vi "Status Section.vi"(8 "error in (no error)":errorcluster, 11 "Node Ptr":T1 format="%.0x") -> (0 "error out":errorcluster)   [LabVIEW 2010, in "RefMem PtByPt Custom Device.lvlib"]
uses:
  RefMem PtByPt Custom Device.lvlib
  <vilib>/NI Veristand/Custom Device API/Custom Device Item Ref.ctl
  <vilib>/NI Veristand/Custom Device API/Custom Device API.lvlib
panel:
  in  "Header":cluster{"Section Name":string}={"Section Name"="Status Section"}
  in  "Description":string
  in  "Name":string
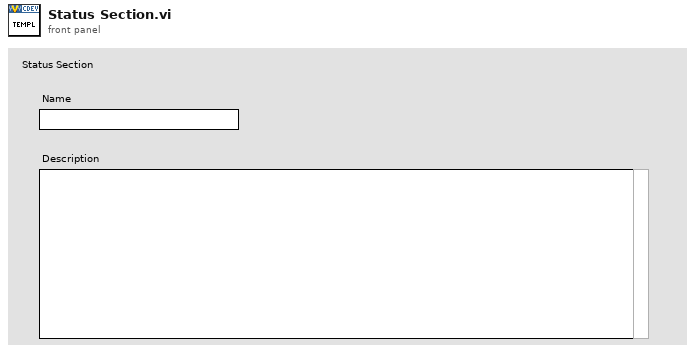
[diagram p1: front panel]
types:
  T1 = typedef "Custom Device API.lvlib/Custom Device Item Ref.ctl" = u64
  T2 = typedef "Custom Device API.lvlib/Custom Device Item Info.ctl" = cluster{"Name":string, "Is Channel":bool, "GUID":string}
  T3 = typedef "Custom Device API.lvlib/Custom Device Commands.ctl" = enum16{"Default", "Item renamed", "Shutdown", "Dynamic button pressed"}
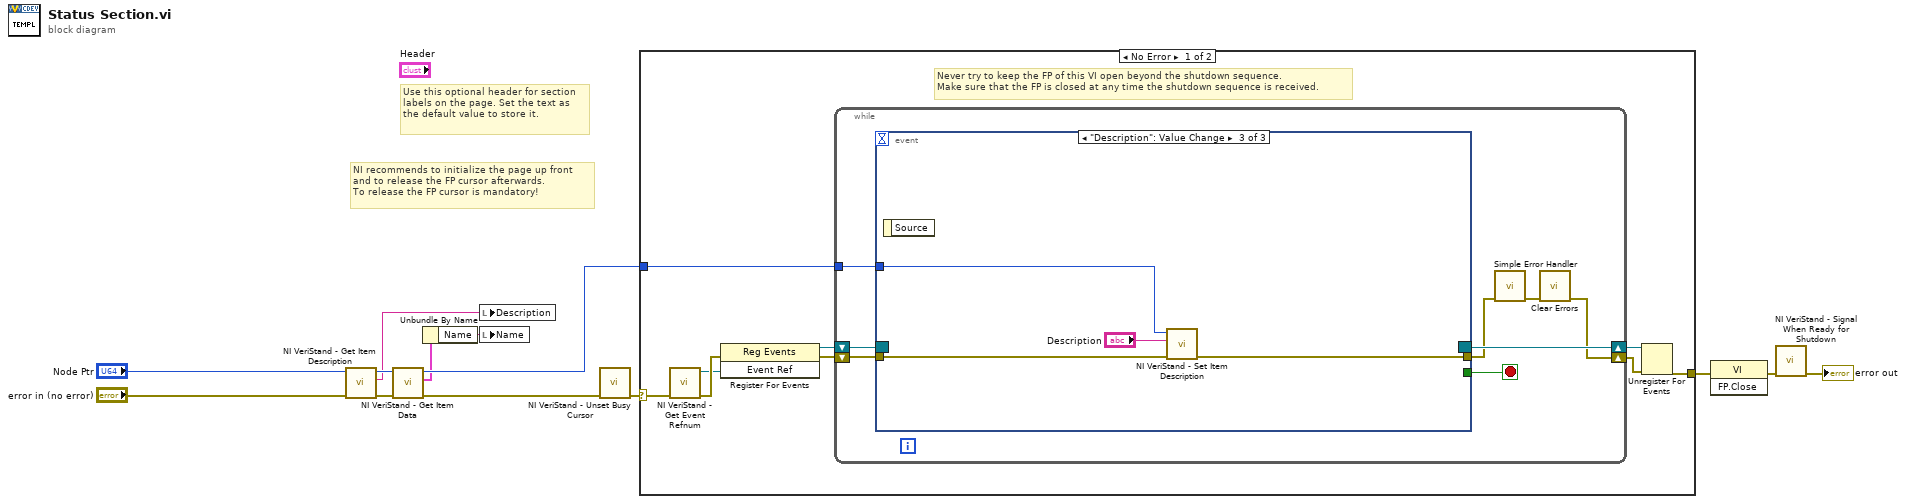
[diagram p0: block diagram]
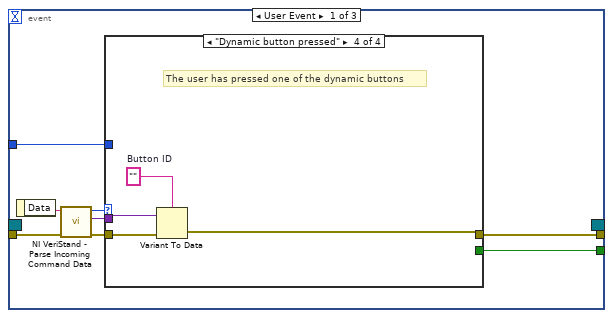
[diagram p2: hidden frame]
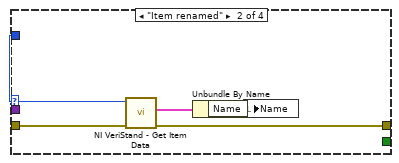
[diagram p4: hidden frame]
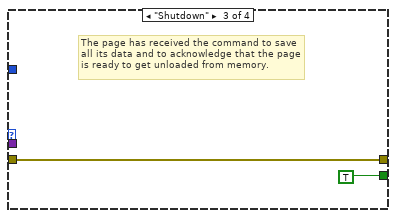
[diagram p5: hidden frame]
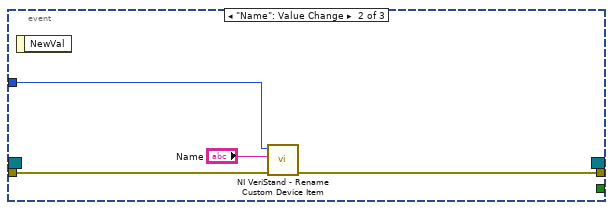
[diagram p6: hidden frame]
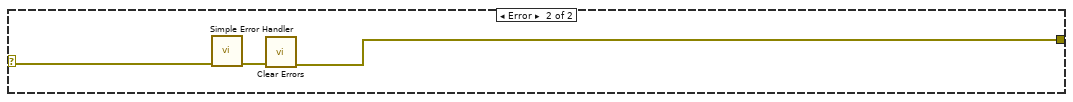
[diagram p7: hidden frame]
diagram:
  # "Use this optional header for section labels on the page. Set the text as the default value to store it."
  # "NI recommends to initialize the page up front\nand to release the FP cursor afterwards.\nTo release the FP cursor is mandatory!"
  n1 = call <vilib>:"NI VeriStand - Get Item Description.vi"("error in (no error)"="error in (no error)", "Item Ref in"="Node Ptr") -> ("error out"=w5:errorcluster, "Description"=w6:string, "Item Ref out"=w7:T1)  [unwired: 7 out]
  n2 = call <vilib>:"NI VeriStand - Get Item Data.vi"("error in (no error)"=w5, "Item Ref in"=w7) -> ("error out"=w10:errorcluster, "Item Info"=w4:T2, "Item Ref out"=w8:T1)  [unwired: 7 out]
  n3 = Unbundle By Name(w4) -> ("Name"=w3:string)
  n4 = local write "Description"(w6) -> ()
  n5 = local write "Name"(w3) -> ()
  n6 = call <vilib>:"NI VeriStand - Unset Busy Cursor.vi"("error in (no error)"=w10) -> ("error out"=w9:errorcluster)  [unwired: 10 out]
  n7 = case shown="No Error" w9 {
    selector: w9 -> [w14 w61]
    tunnel: [w19 w59] -> w13
    tunnel: w8 -> [w15 _]
    frame No Error {
      # "Never try to keep the FP of this VI open beyond the shutdown sequence.\nMake sure that the FP is closed at any time the shutdown sequence is received."
      n8 = call <vilib>:"NI VeriStand - Get Event Refnum.vi"("error in (no error)"=w14) -> ("error out"=w22:errorcluster, "Event Ref"=w18:refnum<user-event>)  [unwired: 9 out]
      n9 = register-events(error in=w22, w18) -> (reference out=w16:refnum<event-registration>, error out=w17:errorcluster)  [unwired: 1 in]
      n10 = while {
        tunnel: w15 -> [w26]
        shift-right: [w23] -> w20
        shift-left: w17 -> [w29]
        shift-right: [w30] -> w21
        shift-left: w16 -> [w28]
        stop <- w27 stop-if-true
        n11 = event shown="[2] \"Description\": Value Change" {
          selector: w28 -> [_ _ _]
          dyn-events: [_ _ _] -> w30
          timeout: _ -> [_ _ _]
          tunnel: w29 -> [w38 w54 w57]
          tunnel: [w34 _ _] -> w27
          tunnel: [w33 w53 w56] -> w25
          tunnel: w26 -> [w32 w52 w58]
          event User Event {
            n12 = event-data() -> ("Data"=w37:string)  [unwired: 1 out]
            n13 = call <vilib>:"NI VeriStand - Parse Incoming Command Data.vi"("error in (no error)"=w38, "Data"=w37) -> ("error out"=w36:errorcluster, "Data"=w31:variant, "Action"=w35:T3)  [unwired: 7 out]
            n14 = case shown="\"Dynamic button pressed\"" w35 {
              tunnel: w36 -> [w39 w44 w45 w50]
              tunnel: [_ _ TRUE _] -> w34
              tunnel: [w39 w41 w45 w47] -> w33
              tunnel: w32 -> [_ w43 _ _]
              tunnel: w31 -> [_ _ _ w49]
              frame "Default", Default {
              }
              frame "Item renamed" {
                n15 = call <vilib>:"NI VeriStand - Get Item Data.vi"("error in (no error)"=w44, "Item Ref in"=w43) -> ("error out"=w41:errorcluster, "Item Info"=w42:T2)  [unwired: 8 out]
                n16 = Unbundle By Name(w42) -> ("Name"=w40:string)
                n17 = local write "Name"(w40) -> ()
              }
              frame "Shutdown" {
                # "The page has received the command to save all its data and to acknowledge that the page is ready to get unloaded from memory."
              }
              frame "Dynamic button pressed" {
                w48 = ""  # Button ID
                # "The user has pressed one of the dynamic buttons"
                n18 = Variant To Data(error in=w50, Variant=w49, type=w48) -> (error out=w47:errorcluster)  [unwired: 1 out]
              }
            }
          }
          event "Name": Value Change {
            n19 = event-data() -> ()  [unwired: 2 out]
            n20 = call <vilib>:"NI VeriStand - Rename Custom Device Item.vi"("error in (no error)"=w54, "New Name"="Name", "Item Ref in"=w52) -> ("error out"=w53:errorcluster)  [unwired: 8 out]
          }
          event "Description": Value Change {
            n21 = event-data() -> ()  [unwired: 2 out]
            n22 = call <vilib>:"NI VeriStand - Set Item Description.vi"("error in (no error)"=w57, "Description"="Description", "Item Ref in"=w58) -> ("error out"=w56:errorcluster)  [unwired: 8 out]
          }
        }
        n23 = call <vilib>:"Simple Error Handler.vi"("error in (no error)"=w25) -> ("error out"=w24:errorcluster)  [unwired: 1 in, 7 out]
        n24 = call <vilib>:"Clear Errors.vi"("error in (no error)"=w24) -> ("error out"=w23:errorcluster)  [unwired: 6 out]
      }
      n25 = Unregister For Events(event registration refnum=w21, error in=w20) -> (error out=w19:errorcluster)
    }
    frame Error {
      n26 = call <vilib>:"Simple Error Handler.vi"("error in (no error)"=w61) -> ("error out"=w60:errorcluster)  [unwired: 1 in, 7 out]
      n27 = call <vilib>:"Clear Errors.vi"("error in (no error)"=w60) -> ("error out"=w59:errorcluster)  [unwired: 6 out]
    }
  }
  n28 = invoke class="VI" method="FP.Close"(error in=w13) -> (error out=w12:errorcluster)  [unwired: 2 in, 2 out]
  n29 = call <vilib>:"NI VeriStand - Signal When Ready for Shutdown.vi"("error in (no error)"=w12) -> ("error out"=→"error out":errorcluster)  [unwired: 10 out]
